vi "get.vi"(8 "error in (no error)":errorcluster, 10 "Key":string, 11 "BundledShapeCache in":refnum<class "BundledShapeCache.lvclass">) -> (0 "error out":errorcluster, 2 "pShape.lvclass":refnum<class "pShape.lvclass">, 3 "BundledShapeCache out":refnum<class "BundledShapeCache.lvclass">)   [LabVIEW 2018, in "BundledShapeCache.lvclass"]
uses:
  BundledShapeCache.lvclass
  Shape Class/pShape.lvclass
  BundledShapeCache.lvclass/BundledShapeCache.ctl
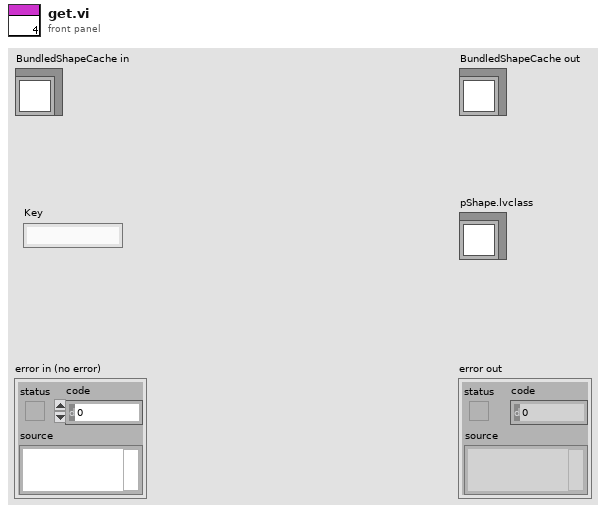
[diagram p1: front panel]
types:
  T1 = cluster{"String":string, "pShape.lvclass":refnum<class "pShape.lvclass">}[]
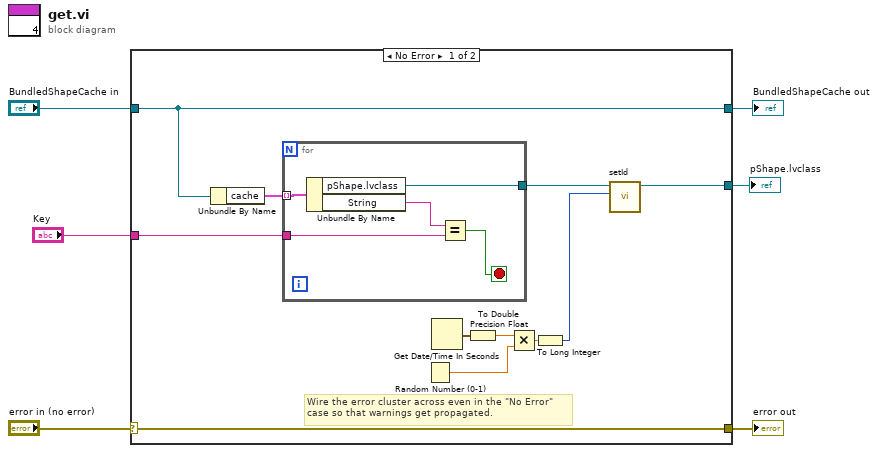
[diagram p0: block diagram]
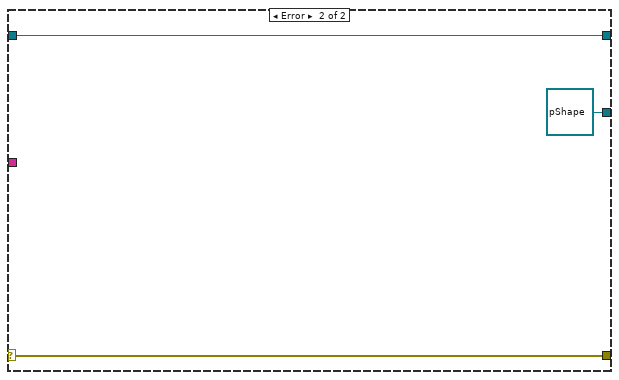
[diagram p2: hidden frame]
diagram:
  n1 = case shown="No Error" "error in (no error)" {
    selector: "error in (no error)" -> [w17 w25]
    tunnel: [w17 w25] -> w5
    tunnel: [w16 w24] -> w3
    tunnel: "BundledShapeCache in" -> [w16 w24]
    tunnel: "Key" -> [w14 _]
    tunnel: [w13 refnum<class "pShape.lvclass"> refnum ("pShape.lvclass")] -> w1
    frame No Error {
      # "Wire the error cluster across even in the \"No Error\"\ncase so that warnings get propagated."
      n2 = Unbundle By Name(w16) -> ("cache"=w15:T1)
      n3 = for {
        tunnel: w15 -> [w22] mode=indexing
        tunnel: w14 -> [w20]
        tunnel: [w18] -> w12
        stop <- w19 stop-if-true
        n4 = Unbundle By Name(w22) -> ("pShape.lvclass"=w18:refnum<class "pShape.lvclass">, "String"=w21:string)
        n5 = Equal?(x=w21, y=w20) -> (x = y?=w19:bool)
      }
      n6 = Random Number (0-1)() -> (number: 0 to 1=w9:dbl)
      n7 = Get Date/Time In Seconds() -> (seconds since 1Jan1904=w11:timestamp)
      n8 = To Double Precision Float(number=w11) -> (double precision float=w10:dbl)
      n9 = Multiply(x=w10, y=w9) -> (x*y=w7:dbl)
      n10 = To Long Integer(number=w7) -> (32bit integer=w8:i32)
      n11 = call-dynamic "setId.vi"("ID"=w8, "pShape in"=w12) -> ("pShape out"=w13:refnum<class "pShape.lvclass">)  [unwired: 8 in, 1 out]
    }
    frame Error {
    }
  }
  "error out" <- w5
  "BundledShapeCache out" <- w3
  "pShape.lvclass" <- w1
